vi "Count Votes.vi"(11 "map in":T1(c390)) -> (2 "Vote Count":T2[](array[typedef]), 3 "map out":T1(c390))   [LabVIEW 2019]
uses:
  Vote Result.ctl
  <vilib>/Utility/miscctls.llb/LVMapReplaceAction.ctl
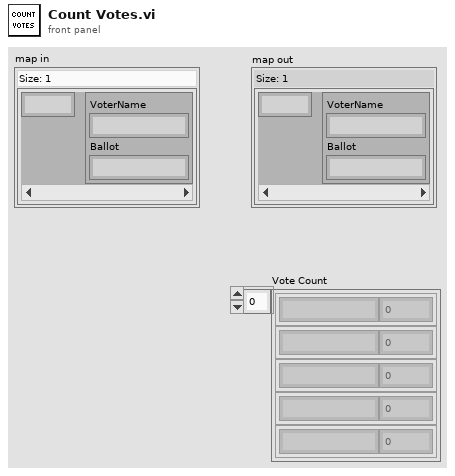
[diagram p1: front panel]
types:
  T1 = map{i32, cluster{"VoterName":string, "Ballot":string}}
  T2 = typedef "Vote Result.ctl" = cluster{"Vote":string, "Count":i32}
  T3 = typedef "LVMapReplaceAction.ctl" = enum32{"Modify Entry only if found", "Add or Modify Entry", "Delete Entry"}
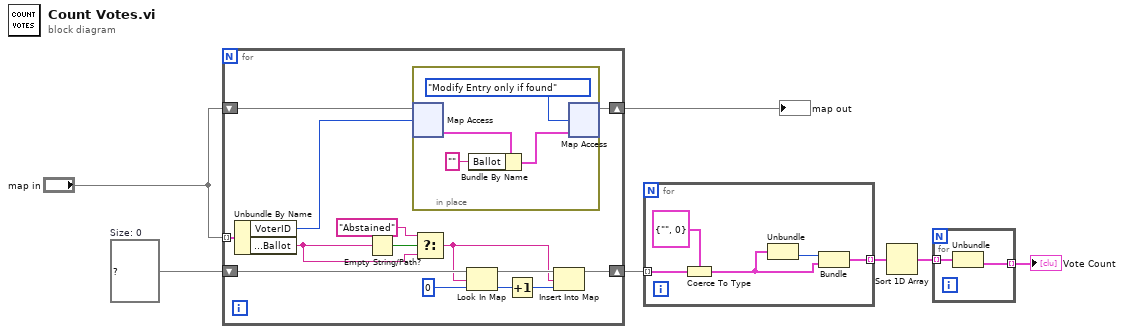
[diagram p0: block diagram]
diagram:
  w6 = map{string, i32} {}  # Size: 0
  n1 = for {
    tunnel: "map in" -> [w20] mode=indexing
    shift-right: [w15] -> w7
    shift-left: w6 -> [w18]
    shift-right: [w13] -> w1
    shift-left: "map in" -> [w14]
    n2 = Unbundle By Name(w20) -> ("VoterID"=w12:i32, "VoterInfo.Ballot"=w10:string)
    n3 = Empty String/Path?(string/path=w10) -> (empty?=w11:bool)
    n4 = in-place {
      n5 = in-place-map #1(w14, w12) -> (w24:cluster{"VoterName":string, "Ballot":string})  [unwired: 1 in, 1 out]
      n6 = Bundle By Name(cluster=w24, "Ballot"="") -> (w22:cluster{"VoterName":string, "Ballot":string})
      n7 = in-place-map #1(w22, LVMapReplaceAction."Modify Entry only if found" ("action")) -> (w13:T1)  [unwired: 2 out]
    }
    n8 = Select(t="Abstained", s=w11, f=w10) -> (s? t:f=w9:string)
    n9 = Look In Map(map=w18, key=w9, default value=0) -> (value=w17:i32)  [unwired: 1 out]
    n10 = Increment(x=w17) -> (x+1=w16:i32)
    n11 = Insert Into Map(map in=w18, key=w9, value=w16) -> (map out=w15:map{string, i32})  [unwired: 2 out]
  }
  "map out" <- w1
  n12 = for {
    tunnel: w7 -> [w27] mode=indexing
    tunnel: [w28] -> w5 mode=indexing
    n13 = Coerce To Type(0:w27, 1:T2 {"Vote"="", "Count"=0} ("Vote Result")) -> (2:w26:T2)
    n14 = Unbundle(w26) -> ("Count"=w29:i32)  [unwired: 1 out]
    n15 = Bundle("Count"=w29, "Vote Result"=w26) -> (w28:cluster{"Count":i32, "Vote Result":T2})  [unwired: 1 in]
  }
  n16 = Sort 1D Array(array=w5) -> (sorted array=w4:cluster{"Count":i32, "Vote Result":T2}[])
  n17 = for {
    tunnel: w4 -> [w31] mode=indexing
    tunnel: [w30] -> w3 mode=indexing
    n18 = Unbundle(w31) -> ("Vote Result"=w30:T2)  [unwired: 1 out]
  }
  "Vote Count" <- w3
